vi "Calculate Frame-to-Frame Head Tail Movement (SubVI).vi"(11 "END Point Cluster Array":T1(array[cluster])) -> (1 "End2":sgl, 2 "Switch?":bool, 3 "End1":sgl)   [LabVIEW 2015]
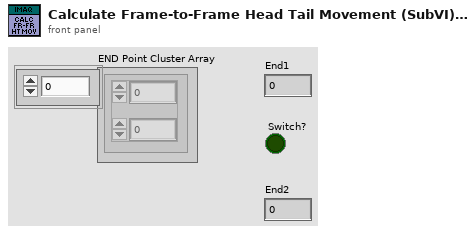
[diagram p1: front panel]
types:
  T1 = cluster{"Numeric Control":sgl, "Numeric Control":sgl}[]
  T2 = cluster{"Numeric Control":sgl, "Numeric Control":sgl}
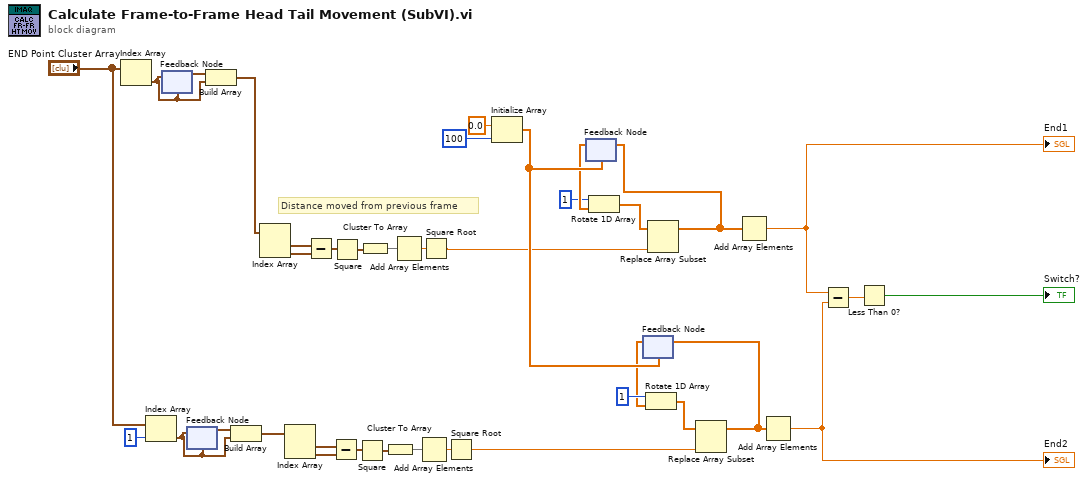
[diagram p0: block diagram]
diagram:
  # "Distance moved from previous frame"
  n1 = Index Array(array="END Point Cluster Array") -> (element=w20:T2)  [unwired: 1 in]
  n2 = Index Array(array="END Point Cluster Array", index=1) -> (element=w12:T2)
  n3 = feedback #1(w20) -> (w5:T2)
  n4 = feedback-in #1(w20) -> ()
  n5 = feedback #2(w12) -> (w13:T2)
  n6 = feedback-in #2(w12) -> ()
  n7 = Build Array(w5, w20) -> (w6:T1)
  n8 = Build Array(w13, w12) -> (w11:T1)
  n9 = Index Array(array=w6) -> (element #1=w7:T2, element #2=w8:T2)  [unwired: 2 in]
  n10 = Index Array(array=w11) -> (element #1=w10:T2, element #2=w9:T2)  [unwired: 2 in]
  n11 = Subtract(x=w7, y=w8) -> (x-y=w3:T2)
  n12 = Subtract(x=w10, y=w9) -> (x-y=w15:T2)
  n13 = Square(x=w3) -> (x^2=w1:T2)
  n14 = Square(x=w15) -> (x^2=w17:T2)
  n15 = Cluster To Array(cluster=w1) -> (array=w4:sgl[])
  n16 = Cluster To Array(cluster=w17) -> (array=w14:sgl[])
  n17 = Add Array Elements(numeric array=w4) -> (sum=w2:sgl)
  n18 = Add Array Elements(numeric array=w14) -> (sum=w16:sgl)
  n19 = Square Root(x=w2) -> (sqrt(x)=w24:sgl)
  n20 = Square Root(x=w16) -> (sqrt(x)=w21:sgl)
  n21 = Initialize Array(sgl 0.0, 100 ("dimension size")) -> (w31:sgl[])
  n22 = feedback #3(w31) -> (w25:sgl[])
  n23 = Rotate 1D Array(1:w25, 2:1 ("n")) -> (0:w26:sgl[])
  n24 = feedback #4(w31) -> (w29:sgl[])
  n25 = Rotate 1D Array(1:w29, 2:1 ("n")) -> (0:w32:sgl[])
  n26 = Replace Array Subset(array=w26, new element=w24) -> (w34:sgl[])  [unwired: 1 in]
  n27 = feedback-in #3(w34) -> ()
  n28 = Replace Array Subset(array=w32, new element=w21) -> (w33:sgl[])  [unwired: 1 in]
  n29 = feedback-in #4(w33) -> ()
  n30 = Add Array Elements(numeric array=w34) -> (sum=w22:sgl)
  "End1" <- w22
  n31 = Add Array Elements(numeric array=w33) -> (sum=w35:sgl)
  "End2" <- w35
  n32 = Subtract(x=w22, y=w35) -> (x-y=w36:sgl)
  n33 = Less Than 0?(x=w36) -> (x < 0?=→"Switch?":bool)
